vi "U8 Array to DBL-Value.vi"(2 "IMU Data Array U8":u8[](array[numeric]), 4 "pos.=lowbyte, pos.+1=highbyte":i32) -> (6 "Data Value (DBL)":dbl)   [LabVIEW 2017]
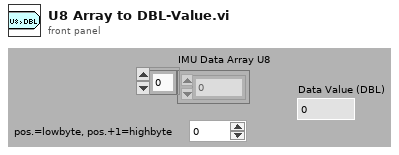
[diagram p1: front panel]
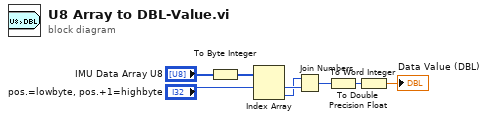
[diagram p0: block diagram]
diagram:
  n1 = To Byte Integer(number="IMU Data Array U8") -> (8bit integer=w8:i8[])
  n2 = Index Array(array=w8, index #1="pos.=lowbyte, pos.+1=highbyte") -> (element #1=w7:i8, element #2=w6:i8)  [unwired: 1 in]
  n3 = Join Numbers(hi=w6, lo=w7) -> ((hi.lo)=w5:u16)
  n4 = To Word Integer(number=w5) -> (16bit integer=w4:i16)
  n5 = To Double Precision Float(number=w4) -> (double precision float=→"Data Value (DBL)":dbl)
